vi "Get Device List.vi"(10 "SQL Server Info":T2, 11 "userID":string) -> (1 "Display Names":string[](array[string]), 2 "Variables":string[](array[string]), 3 "Devices":string[](array[string]))   [LabVIEW 2020]
doc: "This vi list out the devices and variable names and variabl disply names\nInput\n1. Userid\n2.SQL server info\noutput\n1. Array Devices\n2. Variable names\n3. Display names"
uses:
  Shared/MySQL/typedefs/mysql_authentication.ctl
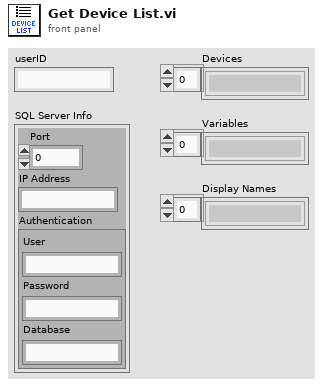
[diagram p1: front panel]
types:
  T1 = typedef "mysql_authentication.ctl" = cluster{"User":string, "Password":string, "Database":string}
  T2 = cluster{"Port":u16, "IP Address":string, "Authentication":T1}
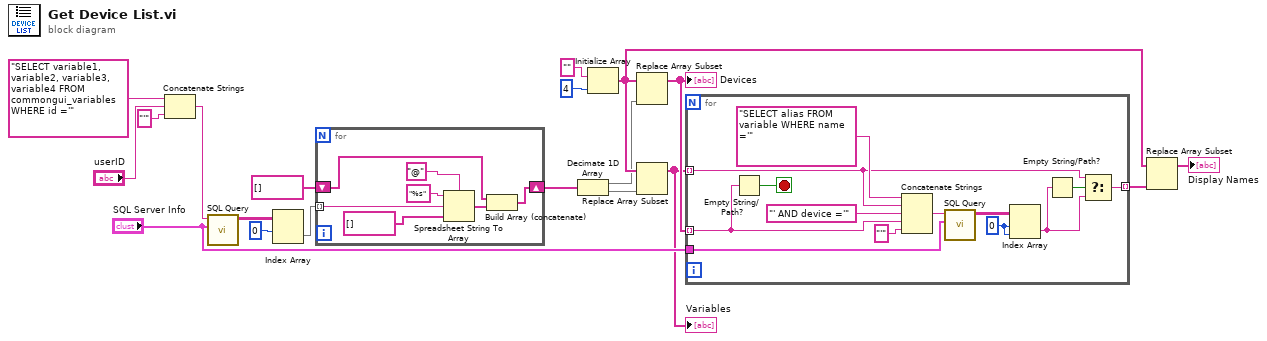
[diagram p0: block diagram]
diagram:
  n1 = Concatenate Strings("SELECT variable1, variable2, variable3, variable4 FROM commongui_variables WHERE id ='", "userID", "'" ("string")) -> (w15:string)
  n2 = call "SQL Query.vi"("SQL Server Info"="SQL Server Info", "Query"=w15) -> ("data"=w2:string[][])  [unwired: 8 in, 1 out]
  n3 = Index Array(array=w2, index (row)=0 ("disabled index (col)")) -> (element=w7:string[])  [unwired: 1 in]
  n4 = for {
    tunnel: w7 -> [w24] mode=indexing
    shift-right: [w21] -> w8
    shift-left: string[] [] -> [w23]
    n5 = Spreadsheet String To Array(delimiter (Tab)="@", format string="%s", spreadsheet string=w24, array type (2D Dbl)=string[] []) -> (array=w22:string[])
    n6 = Build Array (concatenate)(w23, w22) -> (w21:string[])
  }
  n7 = Decimate 1D Array(w8) -> (w11:string[], w12:string[])
  n8 = Initialize Array("", 4 ("dimension size")) -> (w17:string[])
  n9 = Replace Array Subset(array=w17, new element=w11) -> (w14:string[])  [unwired: 1 in]
  "Devices" <- w14
  n10 = Replace Array Subset(array=w17, new element=w12) -> (w13:string[])  [unwired: 1 in]
  "Variables" <- w13
  n11 = for {
    tunnel: w13 -> [w29] mode=indexing
    tunnel: w14 -> [w32] mode=indexing
    tunnel: "SQL Server Info" -> [w35]
    tunnel: [w27] -> w18 mode=indexing
    stop <- w31 stop-if-true
    w34 = 0 ("disabled index (col)")
    n12 = Empty String/Path?(string/path=w32) -> (empty?=w31:bool)
    n13 = Concatenate Strings("SELECT alias FROM variable WHERE name ='", w29, "' AND device ='" ("string"), w32, "'" ("string")) -> (w36:string)
    n14 = call "SQL Query.vi"("SQL Server Info"=w35, "Query"=w36) -> ("data"=w33:string[][])  [unwired: 8 in, 1 out]
    n15 = Index Array(array=w33, index (row)=w34, index (col)=w34) -> (element=w28:string)
    n16 = Empty String/Path?(string/path=w28) -> (empty?=w30:bool)
    n17 = Select(t=w29, s=w30, f=w28) -> (s? t:f=w27:string)
  }
  n18 = Replace Array Subset(array=w17, new element=w18) -> (→"Display Names":string[])  [unwired: 1 in]
